vi "tipshaping.vi"(8 "error in (no error)":errorcluster, 11 "Input":string="-286.640625n,21.171875n,-1.8n,20m,200m") -> (0 "error out":errorcluster, 3 "Output":string="-7.271E-9")   [LabVIEW 2014]
uses:
  <userlib>/Nanonis Prog Interface V5/Nanonis Prog Interface.lvlib
panel:
  in  "Write Markers":bool=TRUE
  in  "milliseconds to wait":u32
  out "size(s)":i32=5
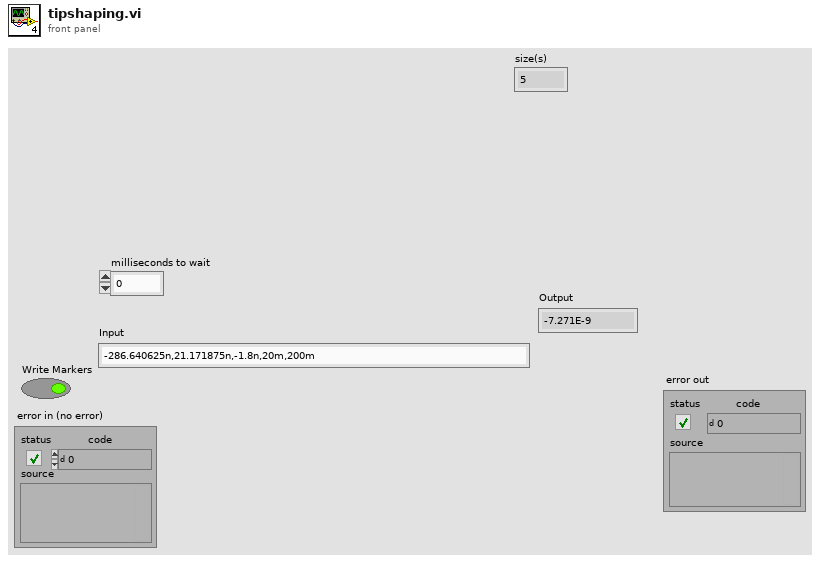
[diagram p1: front panel]
types:
  T1 = cluster{"TipLift":dbl, "Bias Settling Time":dbl, "Lift Height":dbl, "Lift Time 2":dbl, "Lifting Bias":dbl, "Lift Time 1":dbl}
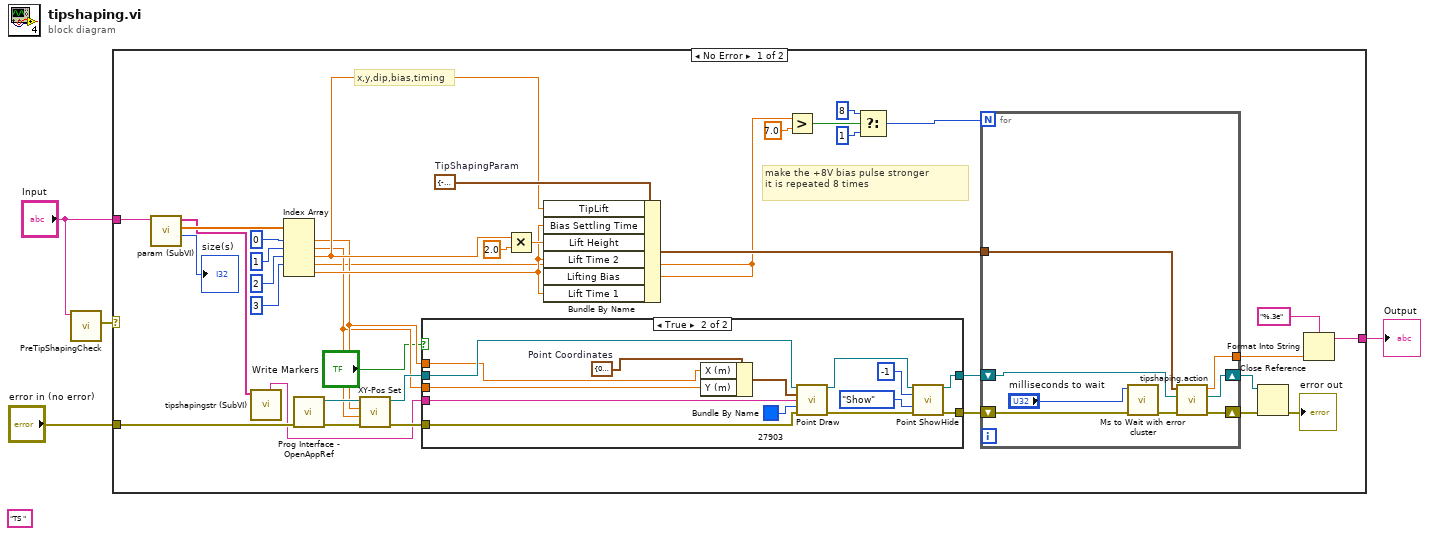
[diagram p0: block diagram]
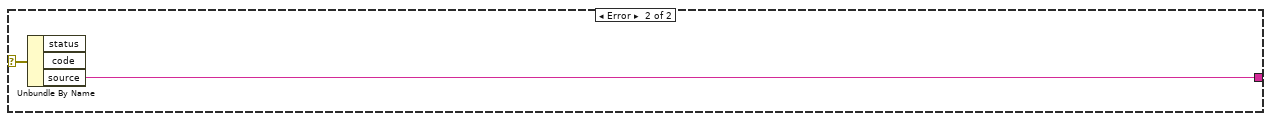
[diagram p3: hidden frame]
diagram:
  (unwired) "TS " ("string")
  n1 = call "PreTipShapingCheck.vi"("Input"="Input") -> ("Error"=w1:errorcluster)  [unwired: 8 in, 2 out]
  n2 = case shown="No Error" w1 {
    selector: w1 -> [_ w67]
    tunnel: [w39 w66] -> w4
    tunnel: "error in (no error)" -> [w32 _]
    tunnel: "Input" -> [w15 _]
    frame No Error {
      w36 = T1 {"TipLift"=-2e-10, "Bias Settling Time"=0.09999999999999999, "Lift Height"=5e-09, "Lift Time 2"=0.2, "Lifting Bias"=2.0, "Lift Time 1"=0.2}  # TipShapingParam
      # "make the +8V bias pulse stronger \nit is repeated 8 times"
      # "x,y,dip,bias,timing"
      n3 = call <userlib>:"param (SubVI).vi"("Input"=w15) -> ("num"=→"size(s)":i32, "parm"=w40:dbl[], "Array"=w16:string[])  [unwired: 8 in]
      n4 = call "tipshapingstr (SubVI).vi"("Array"=w16) -> ("String"=w17:string)  [unwired: 10 in]
      n5 = Index Array(array=w40, index #1=0 ("index"), index #2=1 ("index"), index #3=2 ("index"), index #4=3 ("index")) -> (element #1=w24:dbl, element #2=w23:dbl, element #3=w31:dbl, element #4=w10:dbl, element #5=w28:dbl)  [unwired: 1 in]
      n6 = call <userlib>:"Prog Interface - OpenAppRef.vi"("Error in (no error)"=w32) -> ("Error out"=w33:errorcluster, "Application reference"=w34:refnum<vi>)  [unwired: 5 in]
      n7 = call <userlib>:"XY-Pos Set.vi"("error in (no error)"=w33, "Y (m)"=w23, "X (m)"=w24, "Application ref in"=w34) -> ("error out"=w26:errorcluster, "Application ref out"=w27:refnum<vi>)  [unwired: 4 in]
      n8 = case shown="True" "Write Markers" {
        tunnel: w27 -> [w51 w65]
        tunnel: [w51 w62] -> w14
        tunnel: w26 -> [w50 w64]
        tunnel: [w50 w61] -> w25
        tunnel: w24 -> [_ w54]
        tunnel: w23 -> [_ w53]
        tunnel: w17 -> [_ w52]
        frame False {
        }
        frame True {
          w56 = cluster{"X (m)":sgl, "Y (m)":sgl} {"X (m)"=0.0, "Y (m)"=0.0}  # Point Coordinates
          n9 = Bundle By Name(cluster=w56, "X (m)"=w54, "Y (m)"=w53) -> (w55:cluster{"X (m)":sgl, "Y (m)":sgl})
          n10 = call <userlib>:"Point Draw.vi"("Application ref in"=w65, "Point Coordinates"=w55, "Text"=w52, "Color"=u32 27903, "error in (no error)"=w64) -> ("Application ref out"=w63:refnum<vi>, "error out"=w60:errorcluster)  [unwired: 9 in]
          n11 = call <userlib>:"Point ShowHide.vi"("Application ref in"=w63, "Point index (-1=All points)"=-1, "Show/Hide"=enum16{"Show", "Hide"}."Show", "error in (no error)"=w60) -> ("Application ref out"=w62:refnum<vi>, "error out"=w61:errorcluster)  [unwired: 10 in]
        }
      }
      n12 = Multiply(x=w31, y=2.0) -> (x*y=w30:dbl)
      n13 = Bundle By Name(cluster=w36, "TipLift"=w31, "Bias Settling Time"=w28, "Lift Height"=w30, "Lift Time 2"=w28, "Lifting Bias"=w10, "Lift Time 1"=w28) -> (w35:T1)
      n14 = Greater?(x=w10, y=7.0 ("element")) -> (0:w5:bool)
      n15 = Select(t=8, s=w5, f=1) -> (s? t:f=w8:i32)
      n16 = for {
        N: w8 -> [_]
        tunnel: [w49] -> w38
        tunnel: w35 -> [w48]
        shift-right: [w42] -> w12
        shift-left: w25 -> [w45]
        shift-right: [w43] -> w13
        shift-left: w14 -> [w44]
        n17 = call <userlib>:"Ms to Wait with error cluster.vi"("error in (no error)"=w45, "milliseconds to wait"="milliseconds to wait") -> ("error out"=w47:errorcluster)  [unwired: 4 in, 1 out]
        n18 = call "tipshaping.action.vi"("Error in (no error)"=w47, "Application reference"=w44, "TipShapingParam"=w48) -> ("error out"=w42:errorcluster, "Application ref out"=w43:refnum<vi>, "dz"=w49:sgl)  [unwired: 6 in]
      }
      n19 = Close Reference(reference=w13, error in (no error)=w12) -> (error out=→"error out":errorcluster)
      n20 = Format Into String(format string="%.3e", w38) -> (resulting string=w39:string)  [unwired: 2 in, 1 out]
    }
    frame Error {
      n21 = Unbundle By Name(w67) -> ("source"=w66:string)  [unwired: 2 out]
    }
  }
  "Output" <- w4
